vi "Stop Processes.vi"(11 "VS Inline Async API in":refnum<class "VS Inline Async API.lvclass">) -> (3 "VS Inline Async API out":refnum<class "VS Inline Async API.lvclass">)   [LabVIEW 2015, in "VS Inline Async API.lvlib" / "VS Inline Async API.lvclass"]
uses:
  VS Inline Async API.lvclass
  VS Inline Async API.lvclass/VS Inline Async API.ctl
  <vilib>/NI Veristand/Custom Device Tools/Custom Device Utility Library/Custom Device Utility Library.lvlib
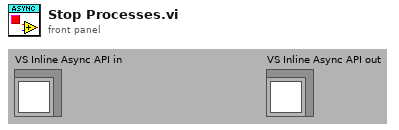
[diagram p1: front panel]
types:
  T1 = enum32{"Bad", "Idle", "Run top level", "Running"}
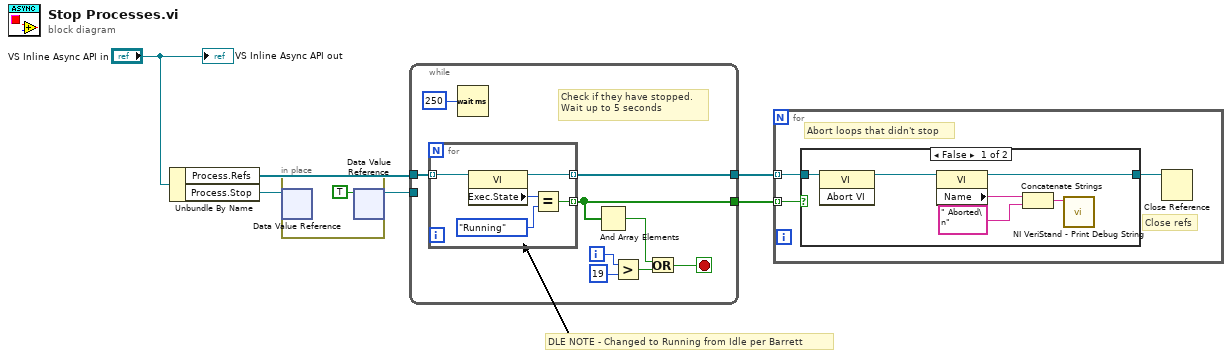
[diagram p0: block diagram]
diagram:
  # "DLE NOTE - Changed to Running from Idle per Barrett"
  n1 = Unbundle By Name("VS Inline Async API in") -> ("Process.Refs"=w4:refnum<vi>[], "Process.Stop"=w2:refnum<data-value>)
  n2 = in-place {
    n3 = in-place-dvr #1(w2) -> ()  [unwired: 2 out]
    n4 = in-place-dvr #1(TRUE ("data value")) -> (w1:refnum<data-value>)  [unwired: 1 out]
  }
  n5 = while {
    tunnel: w4 -> [w15]
    tunnel: [w14] -> w5
    tunnel: [w9] -> w6
    tunnel: w1 -> [_]
    i -> [w12]
    stop <- w13 stop-if-true
    # "Check if they have stopped.\nWait up to 5 seconds"
    n6 = for {
      tunnel: w15 -> [w21] mode=indexing
      tunnel: [w17] -> w9 mode=indexing
      tunnel: [w20] -> w14 mode=indexing
      n7 = property class="VI"(reference=w21) -> (reference out=w20:refnum<vi>, "Exec.State"=w19:T1)  [unwired: 1 in, 1 out]
      n8 = Equal?(x=w19, y=T1."Running") -> (x = y?=w17:bool)
    }
    n9 = Wait (ms)(milliseconds to wait=u32 250) -> ()  [unwired: 1 out]
    n10 = And Array Elements(Boolean array=w9) -> (logical AND=w8:bool)
    n11 = Greater?(x=w12, y=19) -> (0:w10:bool)
    n12 = Or(x=w8, y=w10) -> (x .or. y?=w13:bool)
  }
  n13 = for {
    tunnel: w5 -> [w24] mode=indexing
    tunnel: w6 -> [w23] mode=indexing
    # "Close refs"
    # "Abort loops that didn't stop"
    n14 = case shown="False" w23 {
      tunnel: w24 -> [w30 w31]
      tunnel: [w28 w31] -> w22
      frame False {
        n15 = invoke class="VI" method="Abort VI"(reference=w30) -> (reference out=w29:refnum<vi>)  [unwired: 2 in, 2 out]
        n16 = property class="VI"(reference=w29) -> (reference out=w28:refnum<vi>, "Name"=w27:string)  [unwired: 1 in, 1 out]
        n17 = Concatenate Strings(w27, " Aborted\n" ("string")) -> (w25:string)
        n18 = call <vilib>:"NI VeriStand - Print Debug String.vi"("Message"=w25) -> ()  [unwired: 10 in, 1 out]
      }
      frame True {
      }
    }
    n19 = Close Reference(reference=w22) -> ()  [unwired: 1 in, 1 out]
  }
  "VS Inline Async API out" <- "VS Inline Async API in"
